vi "题目 3.vi"(2 "停止":bool, 3 "温度单位":bool) -> (0 "温度计":dbl(slide) scale=0.0..260.0, 1 "温度":string)   [LabVIEW 2017]
panel:
  # "F"
  # "C"
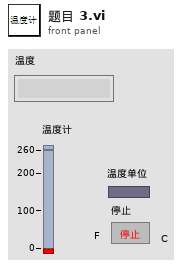
[diagram p1: front panel]
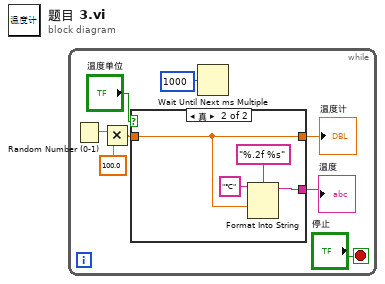
[diagram p0: block diagram]
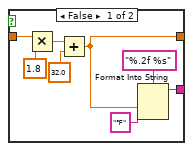
[diagram p2: hidden frame]
diagram:
  n1 = while {
    stop <- "停止" stop-if-true
    n2 = Random Number (0-1)() -> (number: 0 to 1=w2:dbl)
    n3 = Multiply(x=w2, y=100.0) -> (x*y=w7:dbl)
    n4 = case shown="真" "温度单位" {
      tunnel: w7 -> [w13 w18]
      tunnel: [w12 w18] -> w5
      tunnel: [w11 w17] -> w4
      frame False {
        n5 = Multiply(x=w13, y=1.8) -> (x*y=w16:dbl)
        n6 = Add(x=w16, y=32.0) -> (x+y=w12:dbl)
        n7 = Format Into String(format string="%.2f %s" ("格式字符串"), w12, "℉") -> (resulting string=w11:string)  [unwired: 2 in, 1 out]
      }
      frame True {
        n8 = Format Into String(format string="%.2f %s" ("格式字符串"), w18, "℃") -> (resulting string=w17:string)  [unwired: 2 in, 1 out]
      }
    }
    "温度" <- w4
    "温度计" <- w5
    n9 = Wait Until Next ms Multiple(millisecond multiple=u32 1000 ("毫秒倍数")) -> ()  [unwired: 1 out]
  }
